vi "motor_main.vi"() -> ()   [LabVIEW 2020]
uses:
  <vilib>/Instr/_visa.llb/VISA Configure Serial Port (Instr).vi
panel:
  in  "Frenar motor":bool
  out "RPM motor":dbl
  out "Steps/seg Motor":dbl
  in  "n° vueltas":i32=1
  in  "Vel. vuelta":dbl
  in  "Vel. ida":dbl
  in  "Fin":dbl min=0.0 max=180.0 step=0.03
  in  "Inicio":dbl min=0.0 max=180.0 step=0.03
  in  "Auto":bool
  out "Posición":dbl
  in  "Frecuencia\nadquisición\n(ms)":u32=10
  out "backlash":dbl format="%.2f"
  in  "Backlash":bool
  in  "Aceleración (pasos/s^2)":dbl=300.0
  in  "Velocidad (rpm)":dbl=2.0
  out "Grados por paso":dbl
  in  "Switch":u16(ring)=400 items=["200"=200, "400"=400, "600"=600, "800"=800, "1200"=1200, "12000"=12000]
  in  "Adquirir posición":bool
  out "Ángulo":dbl(graph)
  out "Posición":dbl
  in  "Measure":bool
  in  "Home":bool
  out "Status Arduino":bool=TRUE
  in  "Cerrar programa":bool
  in  "Setpoint":dbl min=0.0 max=180.0 step=0.03
  in  "Run":bool
  # "Pruebas"
  # "Configuración General"
  # "Automático"
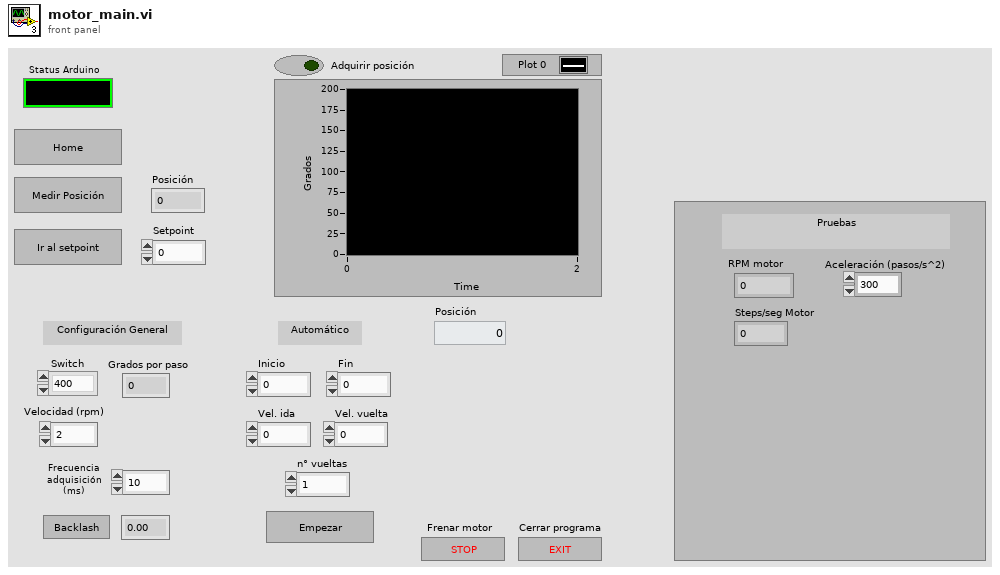
[diagram p1: front panel]
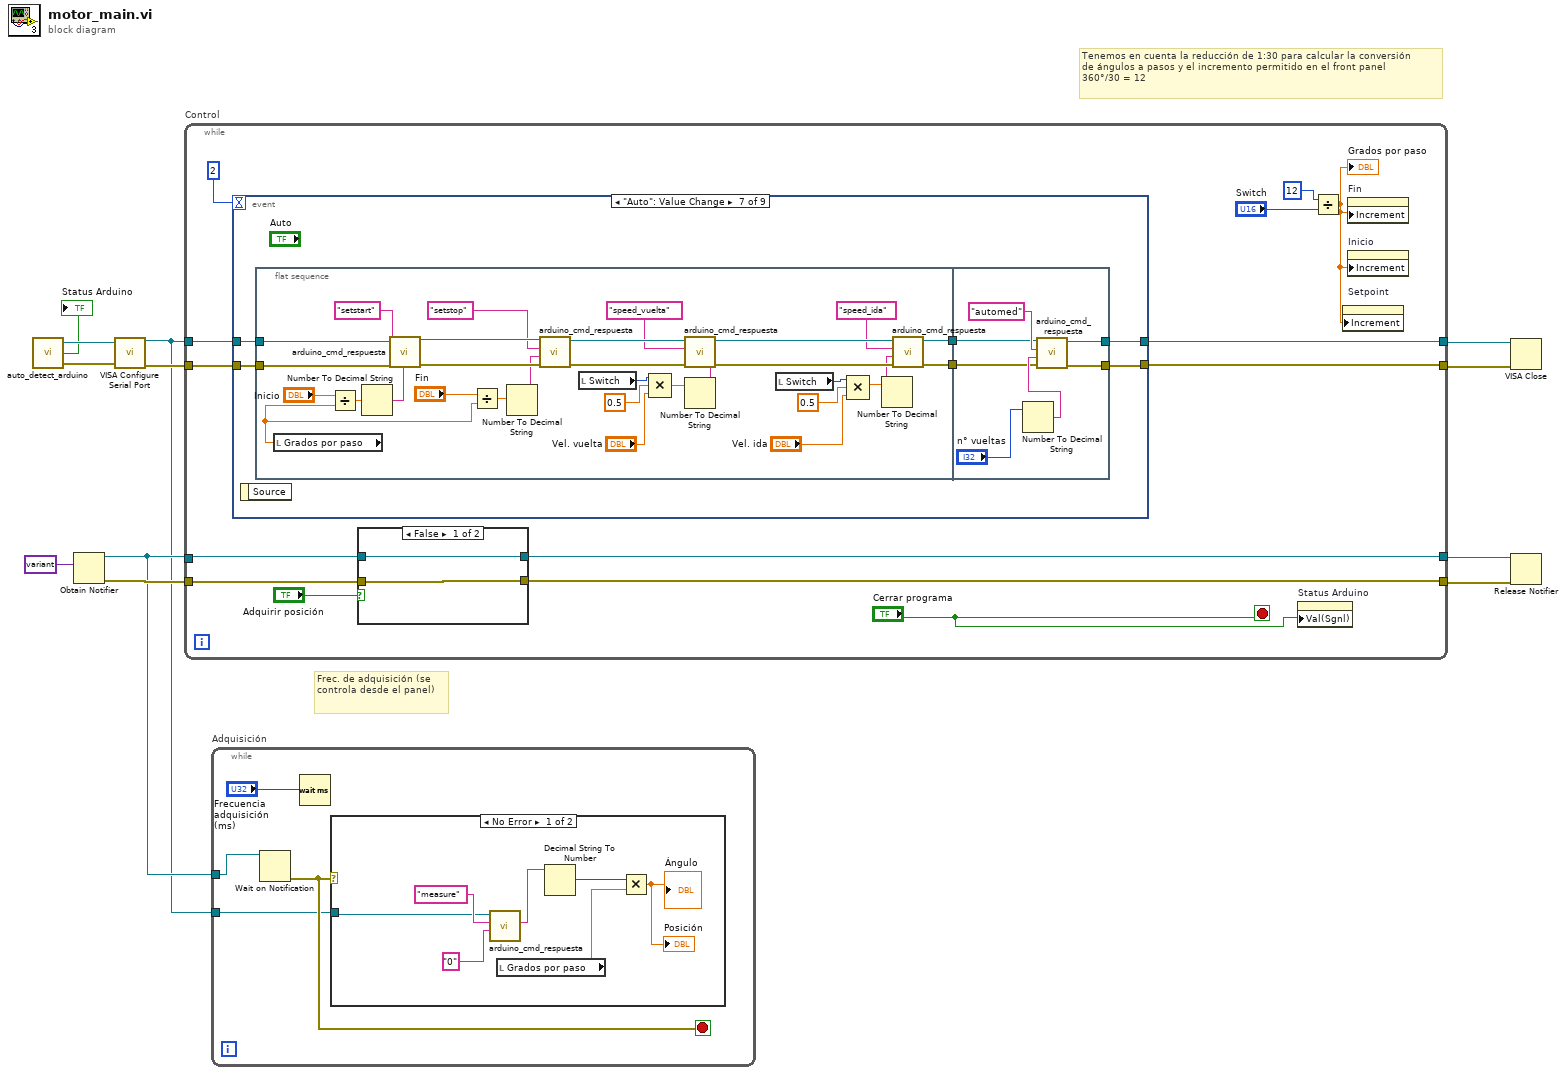
[diagram p0: block diagram]
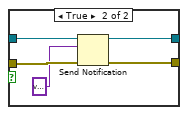
[diagram p3: hidden frame]
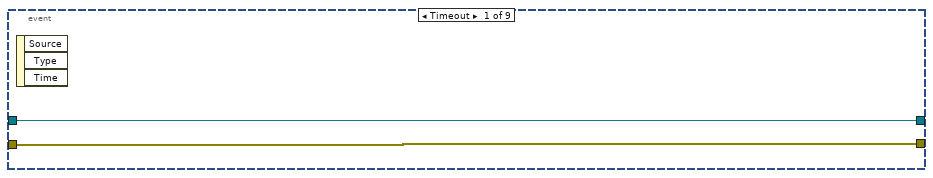
[diagram p4: hidden frame]
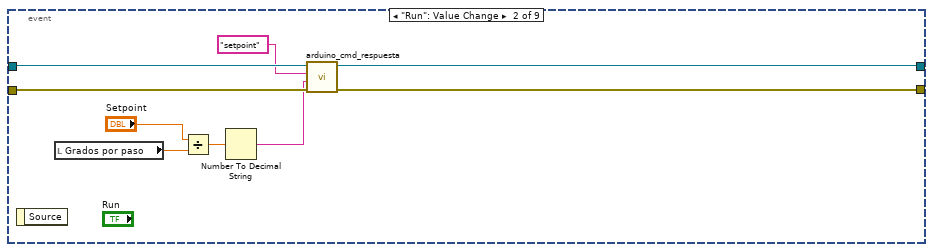
[diagram p5: hidden frame]
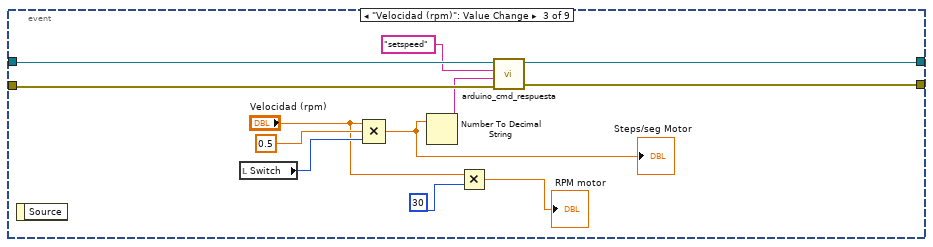
[diagram p6: hidden frame]
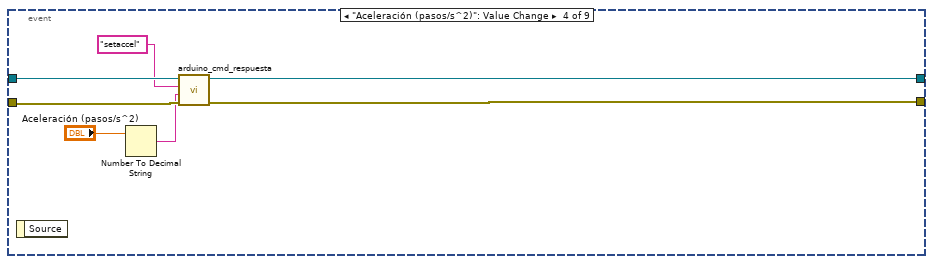
[diagram p7: hidden frame]
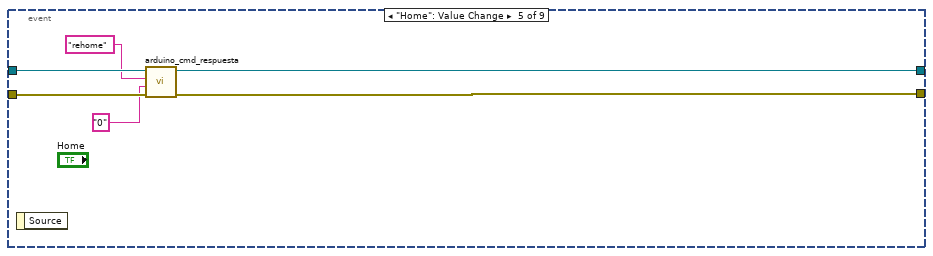
[diagram p8: hidden frame]
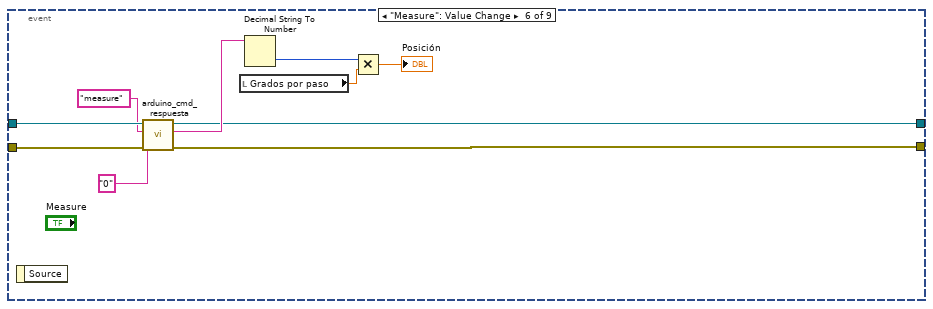
[diagram p9: hidden frame]
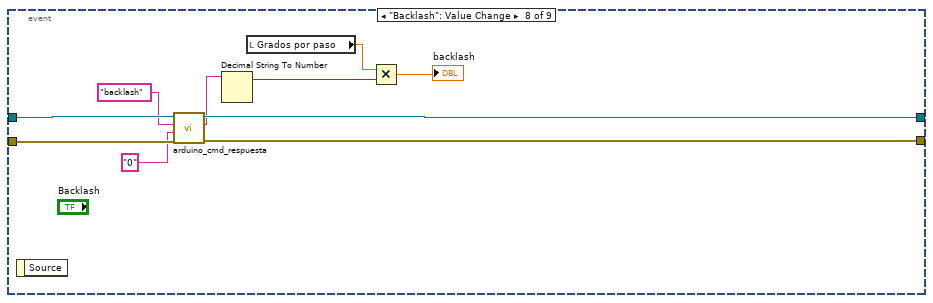
[diagram p10: hidden frame]
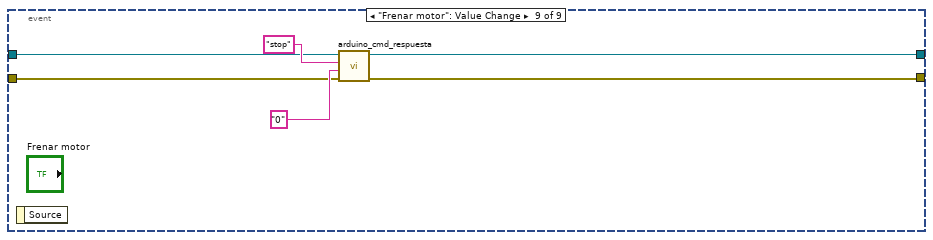
[diagram p11: hidden frame]
diagram:
  # "Tenemos en cuenta la reducción de 1:30 para calcular la conversión\nde ángulos a pasos y el incremento permitido en el front panel\n360°/30 = 12"
  # "Frec. de adquisición (se controla desde el panel)"
  n1 = call "auto_detect_arduino.vi"() -> ("VISA resource name"=w12:refnum<visa-resource-name>, "status"=→"Status Arduino":bool, "error out"=w11:errorcluster)  [unwired: 2 in]
  n2 = Obtain Notifier(notification data type=variant ("element data type")) -> (notifier out=w8:refnum<notifier>, error out=w9:errorcluster)  [unwired: 3 in, 1 out]
  n3 = call-poly "VISA Configure Serial Port"("VISA resource name"=w12, "error in (no error)"=w11) -> ("VISA resource name out"=w1:refnum<visa-resource-name>, "error out"=w2:errorcluster)  [unwired: 12 in]
  n4 = while "Control" {
    tunnel: w1 -> [w26]
    tunnel: w2 -> [w25]
    tunnel: [w24] -> w5
    tunnel: w8 -> [w20]
    tunnel: w9 -> [w19]
    tunnel: [w17] -> w4
    tunnel: [w16] -> w3
    tunnel: [w14] -> w6
    stop <- "Cerrar programa" stop-if-true
    n5 = event shown="[6] \"Auto\": Value Change" {
      selector: _ -> [_ _ _ _ _ _ _ _ _]
      dyn-events: _ -> [_ _ _ _ _ _ _ _ _]
      timeout: 2 -> [_ _ _ _ _ _ _ _ _]
      tunnel: w26 -> [w35 w44 w56 w63 w69 w77 w85 w133 w137]
      tunnel: w25 -> [w34 w43 w55 w62 w68 w78 w84 w131 w136]
      tunnel: [w35 w42 w53 w60 w66 w70 w83 w132 w135] -> w24
      tunnel: [w34 w41 w54 w61 w67 w79 w82 w127 w134] -> w14
      event Timeout {
        n6 = event-data() -> ()  [unwired: 1 in, 3 out]
      }
      event "Run": Value Change {
        n7 = event-data() -> ()  [unwired: 1 in, 1 out]
        n8 = local read "Grados por paso"() -> (w39:dbl)
        n9 = Divide(x="Setpoint", y=w39) -> (x/y=w40:dbl)
        n10 = Number To Decimal String(number=w40) -> (decimal integer string=w37:string)  [unwired: 1 in]
        n11 = call "arduino_cmd_respuesta.vi"("error in (no error)"=w43, "Valor"=w37, "Comando"="setpoint", "VISA resource name in"=w44) -> ("error out"=w41:errorcluster, "VISA resource name out"=w42:refnum<visa-resource-name>)  [unwired: 5 in, 1 out]
      }
      event "Velocidad (rpm)": Value Change {
        n12 = event-data() -> ()  [unwired: 1 in, 1 out]
        n13 = local read "Switch"() -> (w50:u16)
        n14 = Compound Arithmetic op=MULTIPLY("Velocidad (rpm)", 0.5, w50) -> (w46:dbl)
        "Steps/seg Motor" <- w46
        n15 = Number To Decimal String(number=w46) -> (decimal integer string=w52:string)  [unwired: 1 in]
        n16 = Multiply(x="Velocidad (rpm)", y=30) -> (x*y=→"RPM motor":dbl)
        n17 = call "arduino_cmd_respuesta.vi"("error in (no error)"=w55, "Valor"=w52, "Comando"="setspeed", "VISA resource name in"=w56) -> ("error out"=w54:errorcluster, "VISA resource name out"=w53:refnum<visa-resource-name>)  [unwired: 5 in, 1 out]
      }
      event "Aceleración (pasos/s^2)": Value Change {
        n18 = event-data() -> ()  [unwired: 1 in, 1 out]
        n19 = Number To Decimal String(number="Aceleración (pasos/s^2)") -> (decimal integer string=w57:string)  [unwired: 1 in]
        n20 = call "arduino_cmd_respuesta.vi"("error in (no error)"=w62, "Valor"=w57, "Comando"="setaccel", "VISA resource name in"=w63) -> ("error out"=w61:errorcluster, "VISA resource name out"=w60:refnum<visa-resource-name>)  [unwired: 5 in, 1 out]
      }
      event "Home": Value Change {
        n21 = event-data() -> ()  [unwired: 1 in, 1 out]
        n22 = call "arduino_cmd_respuesta.vi"("error in (no error)"=w68, "Valor"="0", "Comando"="rehome", "VISA resource name in"=w69) -> ("error out"=w67:errorcluster, "VISA resource name out"=w66:refnum<visa-resource-name>)  [unwired: 5 in, 1 out]
      }
      event "Measure": Value Change {
        n23 = event-data() -> ()  [unwired: 1 in, 1 out]
        n24 = call "arduino_cmd_respuesta.vi"("error in (no error)"=w78, "Valor"="0", "Comando"="measure", "VISA resource name in"=w77) -> ("error out"=w79:errorcluster, "Respuesta"=w76:string, "VISA resource name out"=w70:refnum<visa-resource-name>)  [unwired: 5 in]
        n25 = local read "Grados por paso"() -> (w73:dbl)
        n26 = Decimal String To Number(string=w76) -> (number=w75:i32)  [unwired: 2 in, 1 out]
        n27 = Multiply(x=w75, y=w73) -> (x*y=→"Posición":dbl)
      }
      event "Auto": Value Change {
        n28 = event-data() -> ()  [unwired: 1 in, 1 out]
        n29 = flat-sequence {
          tunnel: w85 -> [w114]
          tunnel: w84 -> [w113]
          tunnel: [w95] -> w81
          tunnel: [w94] -> w80
          tunnel: [w120] -> w83
          tunnel: [w119] -> w82
          tunnel: w81 -> [w118]
          tunnel: w80 -> [w117]
          frame #0 {
            n30 = local read "Grados por paso"() -> (w104:dbl)
            n31 = Divide(x="Inicio", y=w104) -> (x/y=w112:dbl)
            n32 = Number To Decimal String(number=w112) -> (decimal integer string=w110:string)  [unwired: 1 in]
            n33 = call "arduino_cmd_respuesta.vi"("error in (no error)"=w113, "Valor"=w110, "Comando"="setstart", "VISA resource name in"=w114) -> ("error out"=w115:errorcluster, "VISA resource name out"=w116:refnum<visa-resource-name>)  [unwired: 5 in, 1 out]
            n34 = Divide(x="Fin", y=w104) -> (x/y=w108:dbl)
            n35 = Number To Decimal String(number=w108) -> (decimal integer string=w105:string)  [unwired: 1 in]
            n36 = call "arduino_cmd_respuesta.vi"("error in (no error)"=w115, "Valor"=w105, "Comando"="setstop", "VISA resource name in"=w116) -> ("error out"=w102:errorcluster, "VISA resource name out"=w103:refnum<visa-resource-name>)  [unwired: 5 in, 1 out]
            n37 = local read "Switch"() -> (w93:u16)
            n38 = Compound Arithmetic op=MULTIPLY(w93, 0.5, "Vel. vuelta") -> (w90:dbl)
            n39 = Number To Decimal String(number=w90) -> (decimal integer string=w99:string)  [unwired: 1 in]
            n40 = call "arduino_cmd_respuesta.vi"("error in (no error)"=w102, "Valor"=w99, "Comando"="speed_vuelta", "VISA resource name in"=w103) -> ("error out"=w100:errorcluster, "VISA resource name out"=w101:refnum<visa-resource-name>)  [unwired: 5 in, 1 out]
            n41 = local read "Switch"() -> (w88:u16)
            n42 = Compound Arithmetic op=MULTIPLY(w88, 0.5, "Vel. ida") -> (w89:dbl)
            n43 = Number To Decimal String(number=w89) -> (decimal integer string=w98:string)  [unwired: 1 in]
            n44 = call "arduino_cmd_respuesta.vi"("error in (no error)"=w100, "Valor"=w98, "Comando"="speed_ida", "VISA resource name in"=w101) -> ("error out"=w94:errorcluster, "VISA resource name out"=w95:refnum<visa-resource-name>)  [unwired: 5 in, 1 out]
          }
          frame #1 {
            n45 = Number To Decimal String(number="n° vueltas") -> (decimal integer string=w121:string)  [unwired: 1 in]
            n46 = call "arduino_cmd_respuesta.vi"("error in (no error)"=w117, "Valor"=w121, "Comando"="automed", "VISA resource name in"=w118) -> ("error out"=w119:errorcluster, "VISA resource name out"=w120:refnum<visa-resource-name>)  [unwired: 5 in, 1 out]
          }
        }
      }
      event "Backlash": Value Change {
        n47 = event-data() -> ()  [unwired: 1 in, 1 out]
        n48 = call "arduino_cmd_respuesta.vi"("error in (no error)"=w131, "Valor"="0", "Comando"="backlash", "VISA resource name in"=w133) -> ("error out"=w127:errorcluster, "Respuesta"=w130:string, "VISA resource name out"=w132:refnum<visa-resource-name>)  [unwired: 5 in]
        n49 = Decimal String To Number(string=w130) -> (offset past number=w126:i32)  [unwired: 2 in, 1 out]
        n50 = local read "Grados por paso"() -> (w125:dbl)
        n51 = Multiply(x=w125, y=w126) -> (x*y=→"backlash":dbl)
      }
      event "Frenar motor": Value Change {
        n52 = event-data() -> ()  [unwired: 1 in, 1 out]
        n53 = call "arduino_cmd_respuesta.vi"("error in (no error)"=w136, "Valor"="0", "Comando"="stop", "VISA resource name in"=w137) -> ("error out"=w134:errorcluster, "VISA resource name out"=w135:refnum<visa-resource-name>)  [unwired: 5 in, 1 out]
      }
    }
    n54 = case shown="False" "Adquirir posición" {
      tunnel: w20 -> [w27 w33]
      tunnel: w19 -> [w28 w30]
      tunnel: [w27 w32] -> w17
      tunnel: [w28 w31] -> w16
      frame False {
      }
      frame True {
        n55 = Send Notification(notification=variant, notifier=w33, error in (no error)=w30) -> (notifier out=w32:refnum<notifier>, error out=w31:errorcluster)
      }
    }
    n56 = property on="Status Arduino" class="Bool (strict)"("Val(Sgnl)"="Cerrar programa") -> ()  [unwired: 2 in, 2 out]
    n57 = Divide(x=12, y="Switch") -> (x/y=w15:dbl)
    "Grados por paso" <- w15
    n58 = property on="Setpoint" class="DigNum (strict)"("Increment"=w15) -> ()  [unwired: 2 in, 2 out]
    n59 = property on="Fin" class="DigNum (strict)"("Increment"=w15) -> ()  [unwired: 2 in, 2 out]
    n60 = property on="Inicio" class="DigNum (strict)"("Increment"=w15) -> ()  [unwired: 2 in, 2 out]
  }
  n61 = while "Adquisición" {
    tunnel: w8 -> [w143]
    tunnel: w1 -> [w140]
    stop <- w141 stop-if-true
    n62 = Wait on Notification(notifier=w143) -> (error out=w141:errorcluster)  [unwired: 3 in, 3 out]
    n63 = Wait (ms)(milliseconds to wait="Frecuencia\nadquisición\n(ms)") -> ()  [unwired: 1 out]
    n64 = case shown="No Error" w141 {
      tunnel: w140 -> [w144 _]
      frame No Error {
        n65 = call "arduino_cmd_respuesta.vi"("Valor"="0", "Comando"="measure", "VISA resource name in"=w144) -> ("Respuesta"=w148:string)  [unwired: 6 in, 2 out]
        n66 = local read "Grados por paso"() -> (w150:dbl)
        n67 = Decimal String To Number(string=w148) -> (number=w149:i32)  [unwired: 2 in, 1 out]
        n68 = Multiply(x=w149, y=w150) -> (x*y=→"Ángulo" →"Posición":dbl)
      }
      frame Error {
      }
    }
  }
  n69 = VISA Close(VISA resource name=w5, error in (no error)=w6) -> ()  [unwired: 1 out]
  n70 = Release Notifier(notifier=w4, error in (no error)=w3) -> ()  [unwired: 1 in, 3 out]
